vi "Передатчик(связь с USRP ).vi"() -> ()   [LabVIEW 2013]
uses:
  <vilib>/Analysis/baseanly.llb/A x B.vi
  <vilib>/Analysis/baseanly.llb/Real A x B.vi
  <vilib>/Analysis/Matrix/Numeric/Conversions/Array To Matrix.vi
  <vilib>/Analysis/Matrix/Numeric/Conversions/Array To Matrix - RA.vi
  <instrlib>/niUSRP/niUSRP Write Tx Data (CDB).vi
panel:
  in  "Остановить":bool
  in  "Обновить":bool
  in  "gain":dbl format="%#_6f"
  in  "amplitudes 2":dbl[](array[slide])=[2.3636363636363638, 0.4545454545454546, 0.4545454545454546, 0.5, 0.5, 0.5, 0.5, 0.5, 0.5, 0.5, 0.5, 0.5, 0.5, 0.5, 0.5, 0.5, 0.5, 0.5, 0.5, 0.5, 0.5, 0.5, 0.5, 0.5, 0.5, 0.5, 0.5, 0.5, 0.5, 0.5, 0.5, 0.5, 0.5, 0.5, 0.5, 0.4545454545454546, 0.4545454545454546, 0.4545454545454546, 0.4545454545454546, 0.4545454545454546, 0.4545454545454546, 0.4545454545454546, 0.4545454545454546, 0.4545454545454546, 0.4545454545454546, 0.4545454545454546, 0.4545454545454546, 0.4545454545454546, 0.4545454545454546, 0.4545454545454546, 0.4545454545454546, 0.4545454545454546, 0.4545454545454546, 0.4545454545454546, 0.4545454545454546, 0.4545454545454546, 0.4545454545454546, 0.4545454545454546, 0.4545454545454546, 0.4545454545454546, 0.4545454545454546, 0.4545454545454546, 0.4545454545454546, 0.4545454545454546] scale=0.0..4.0
  out "transmitted bits":bool[][](array[boolean])
  in  "carrier freq.":dbl=850000000.0 format="%#_6p"
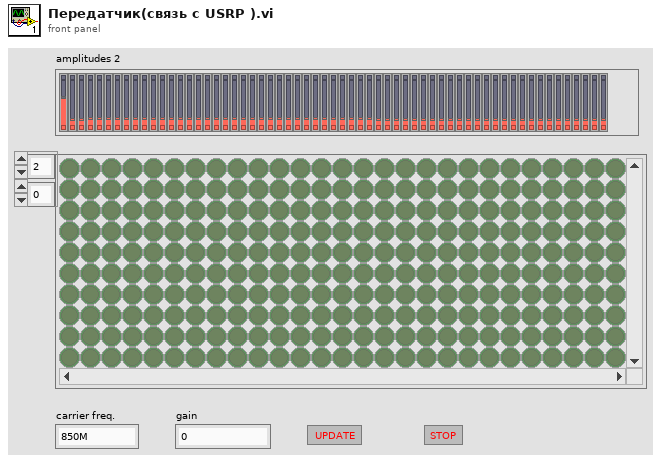
[diagram p1: front panel]
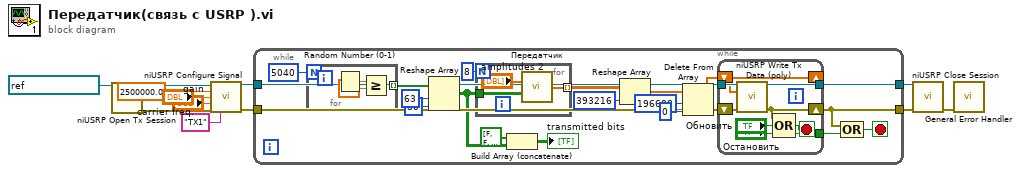
[diagram p0: block diagram]
diagram:
  n1 = call <instrlib>:"niUSRP Open Tx Session.vi"("device names"=refnum<k15> "192.168.10.2") -> ("session handle out"=w12:refnum<k15>, "error out"=w11:errorcluster)  [unwired: 13 in]
  n2 = call <instrlib>:"niUSRP Configure Signal.vi"("session handle"=w12, "IQ rate"=2500000.0, "carrier frequency"="carrier freq.", "gain"="gain", "error in (no error)"=w11, "active antenna"="TX1") -> ("session handle out"=w3:refnum<k15>, "error out"=w2:errorcluster)  [unwired: 5 in, 3 out]
  n3 = while {
    tunnel: [w23] -> w5
    tunnel: [w17] -> w4
    tunnel: w3 -> [w21]
    tunnel: w2 -> [w20]
    stop <- w19 stop-if-true
    n4 = for {
      N: 5040 -> [_]
      tunnel: [w44] -> w22 mode=indexing
      n5 = Random Number (0-1)() -> (number: 0 to 1=w46:dbl)
      n6 = Greater Or Equal?(x=w46, y=0.5) -> (x >= y?=w44:bool)
    }
    n7 = Reshape Array(w22, 63 ("dimension size"), 80 ("dimension size")) -> (w14:bool[][])
    n8 = for {
      N: 8 -> [_]
      tunnel: w14 -> [w43]
      tunnel: [w42] -> w28 mode=indexing
      n9 = call "Передатчик.vi"("Амплитуды\nканала трафика"="amplitudes 2", "Биты для \nпередачи"=w43) -> ("x + iy"=w42:cdb[])  [unwired: 13 in]
    }
    n10 = Build Array (concatenate)(bool[] [FALSE, FALSE, FALSE, FALSE, FALSE, FALSE, FALSE, FALSE, FALSE, FALSE, FALSE, FALSE, FALSE, FALSE, FALSE, FALSE, FALSE, FALSE, FALSE, FALSE, FALSE, FALSE, FALSE, FALSE, FALSE, FALSE, FALSE, FALSE, FALSE, FALSE, FALSE, FALSE, FALSE, FALSE, FALSE, FALSE, FALSE, FALSE, FALSE, FALSE, FALSE, FALSE, FALSE, FALSE, FALSE, FALSE, FALSE, FALSE, FALSE, FALSE, FALSE, FALSE, FALSE, FALSE, FALSE, FALSE, FALSE, FALSE, FALSE, FALSE, FALSE, FALSE, FALSE, FALSE, FALSE, FALSE, FALSE, FALSE, FALSE, FALSE, FALSE, FALSE, FALSE, FALSE, FALSE, FALSE, FALSE, FALSE, FALSE, FALSE] ("Array"), w14) -> (→"transmitted bits":bool[][])
    n11 = Reshape Array(w28, 393216 ("dimension size")) -> (w30:cdb[])
    n12 = Delete From Array(array=w30, length=196608, index=0) -> (array with subset deleted=w16:cdb[])  [unwired: 1 out]
    n13 = while {
      shift-right: [w34] -> w17
      shift-left: w20 -> [w39]
      tunnel: [w37] -> w23
      tunnel: w21 -> [w36]
      tunnel: ["Остановить"] -> w18
      shift-right: [w33] -> _
      shift-left: w16 -> [w33]
      stop <- w40 stop-if-true
      n14 = call-poly <instrlib>:"niUSRP Write Tx Data (poly).vi"("session handle"=w36, "data"=w33, "error in (no error)"=w39) -> ("session handle out"=w37:refnum<k15>, "error out"=w34:errorcluster)  [unwired: 11 in]
      n15 = Compound Arithmetic op=OR(w34, "Обновить", "Остановить") -> (w40:bool)
    }
    n16 = Compound Arithmetic op=OR(w17, w18) -> (w19:bool)
  }
  n17 = call <instrlib>:"niUSRP Close Session.vi"("session handle"=w5, "error in (no error)"=w4) -> ("error out"=w1:errorcluster)  [unwired: 13 in]
  n18 = call <vilib>:"General Error Handler.vi"("error in (no error)"=w1) -> ()  [unwired: 10 in, 5 out]
